vi "Stringhandling (SubVI).vi"(0 "Slide (Eingang)":refnum<vi>, 1 "Füllstand Lesepuffer (Eingang)":i32, 2 "Datei COM (Eingang)":refnum<file>, 3 "VISA-Referenz (Eingang)":refnum<visa-resource-name>, 4 "MessFrequenz [Hz] (Eingang)":dbl, 5 "Bytes at Port":u32, 6 "Datei LV (Eingang)":refnum<file>, 7 "Fehler (Eingang, kein Fehler)":errorcluster, 8 "Cyclecounter (Eingang)":i32, 9 "Rolle[Hz] (Eingang)":dbl, 10 "Temp[°C] (Eingang)":dbl, 11 "AFR (Eingang)":dbl, 12 "String (Eingang)":string, 13 "Zündung [Hz] (Eingang)":dbl) -> (14 "Lesepuffer":string="\n", 16 "Füllstand Lesepuffer (Ausgang)":i32, 17 "String (Ausgang)":string, 18 "Temp[°C] (Ausgang)":dbl, 19 "AFR (Ausgang)":dbl, 20 "VISA-Referenz (Ausgang)":refnum<visa-resource-name>, 21 "Zündung [Hz] (Ausgang)":dbl, 23 "Rolle [Hz] (Ausgang)":dbl, 24 "Messfrequenz [Hz] (Ausgang)":dbl, 25 "Cyclecounter (Ausgang)":i32, 27 "Fehler (Ausgang)":errorcluster)   [LabVIEW 2014]
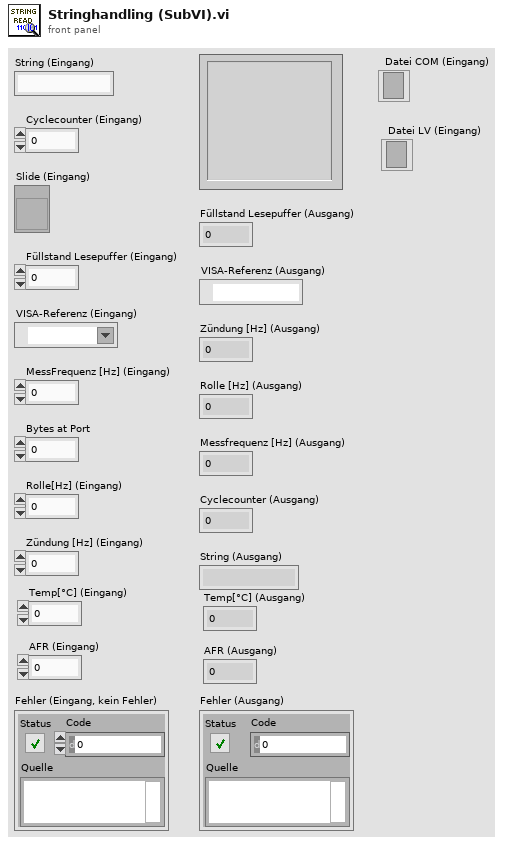
[diagram p1: front panel]
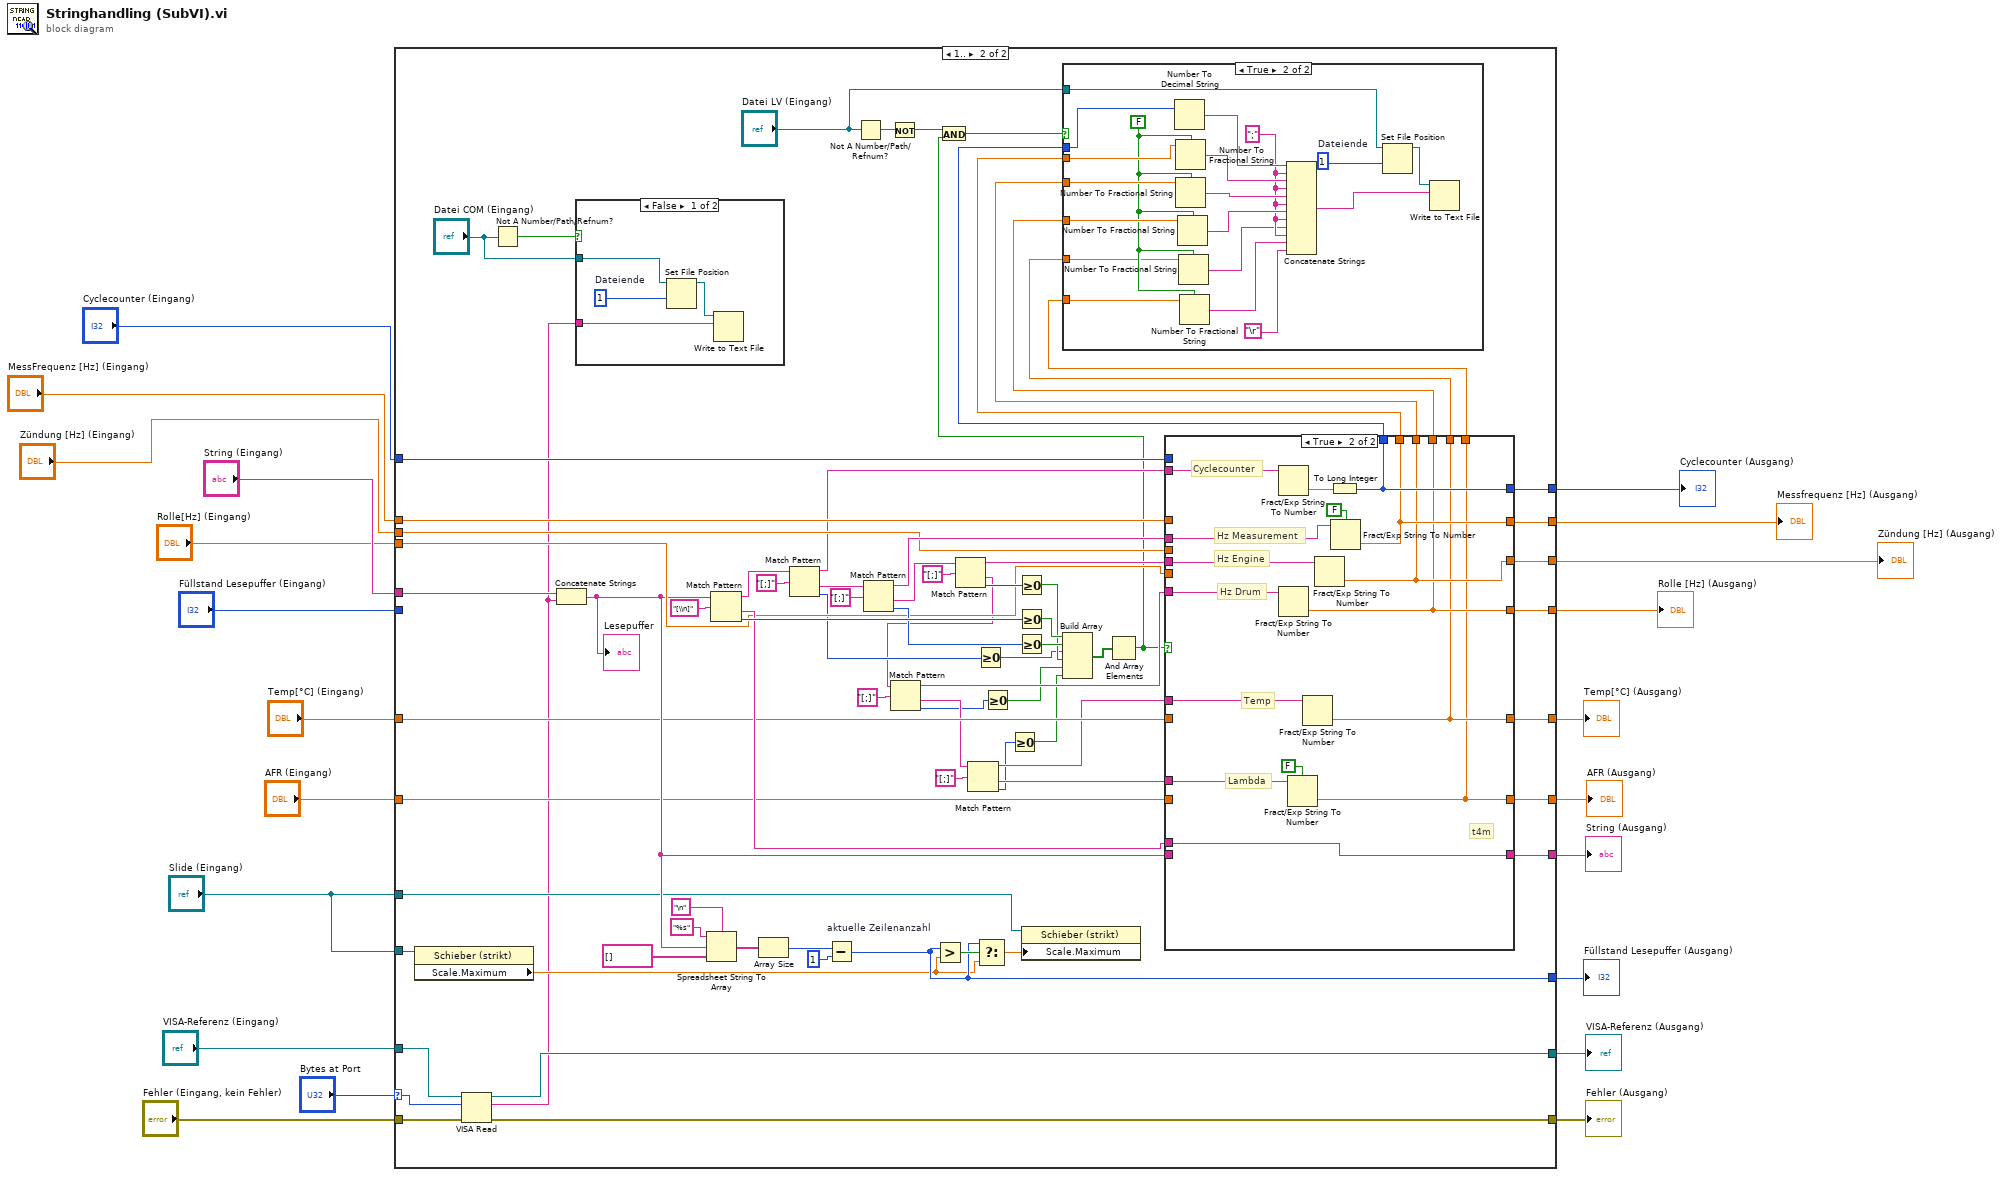
[diagram p0: block diagram]
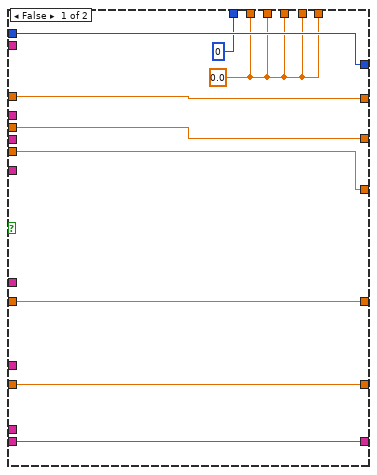
[diagram p5: hidden frame]
diagram:
  n1 = case shown="1.." "Bytes at Port" {
    selector: "Bytes at Port" -> [_ w104]
    tunnel: [w26 w99] -> w14
    tunnel: [w25 w100] -> w19
    tunnel: [w30 w101] -> w12
    tunnel: [w31 w98] -> w11
    tunnel: "String (Eingang)" -> [w32 w97]
    tunnel: [w32 w95] -> w6
    tunnel: "Zündung [Hz] (Eingang)" -> [w31 w88]
    tunnel: "Rolle[Hz] (Eingang)" -> [w30 w87]
    tunnel: [w27 w86] -> w15
    tunnel: "MessFrequenz [Hz] (Eingang)" -> [w27 w85]
    tunnel: "Füllstand Lesepuffer (Eingang)" -> [w29 _]
    tunnel: [w29 w68] -> w13
    tunnel: [w28 w74] -> w16
    tunnel: "Cyclecounter (Eingang)" -> [w28 w73]
    tunnel: "VISA-Referenz (Eingang)" -> [w25 w65]
    tunnel: "Fehler (Eingang, kein Fehler)" -> [w26 w64]
    tunnel: "Slide (Eingang)" -> [_ w63]
    tunnel: "Slide (Eingang)" -> [_ w62]
    tunnel: "Temp[°C] (Eingang)" -> [w24 w61]
    tunnel: [w24 w60] -> w3
    tunnel: [w23 w59] -> w2
    tunnel: "AFR (Eingang)" -> [w23 w58]
    frame 0, Default {
      # "No data in from serial port - Nothing to do."
    }
    frame 1.. {
      n2 = property on="Eigenschaftsknoten" class="Schieber (strikt)"(reference=w63) -> ("Scale.Maximum"=w67:dbl)  [unwired: 1 in, 2 out]
      n3 = VISA Read(VISA resource name=w65, byte count=w104, error in (no error)=w64) -> (VISA resource name out=w100:refnum<visa-resource-name>, read buffer=w45:string, error out=w99:errorcluster)  [unwired: 1 out]
      n4 = Not A Number/Path/Refnum?(number/path/refnum="Datei COM (Eingang)") -> (NaN/Path/Refnum?=w46:bool)
      n5 = Concatenate Strings(w97, w45) -> (w70:string)
      "Lesepuffer" <- w70
      n6 = case shown="False" w46 {
        tunnel: w45 -> [w130 _]
        tunnel: "Datei COM (Eingang)" -> [w129 _]
        frame False {
          w132 = 1  # Dateiende
          n7 = Set File Position(refnum=w129, from (0:start)=w132) -> (refnum out=w131:refnum<file>)  [unwired: 2 in, 1 out]
          n8 = Write to Text File(file (use dialog)=w131, text=w130) -> ()  [unwired: 2 in, 3 out]
        }
        frame True {
        }
      }
      n9 = Spreadsheet String To Array(delimiter (Tab)="\n" ("regular expression"), format string="%s" ("regular expression"), spreadsheet string=w70, array type (2D Dbl)=string[] [] ("Array 2")) -> (array=w79:string[])
      n10 = Match Pattern(string=w70, regular expression="[\\n]") -> (before substring=w77:string, after substring=w96:string, offset past match=w108:i32)  [unwired: 1 in, 1 out]
      n11 = Array Size(array=w79) -> (size(s)=w83:i32)
      n12 = Match Pattern(string=w77, regular expression="[;]") -> (before substring=w75:string, after substring=w76:string, offset past match=w72:i32)  [unwired: 1 in, 1 out]
      n13 = Subtract "aktuelle Zeilenanzahl"(x=w83, y=1) -> (x-y=w68:i32)
      n14 = Not A Number/Path/Refnum?(number/path/refnum="Datei LV (Eingang)") -> (NaN/Path/Refnum?=w34:bool)
      n15 = Match Pattern(string=w76, regular expression="[;]") -> (before substring=w103:string, after substring=w106:string, offset past match=w93:i32)  [unwired: 1 in, 1 out]
      n16 = Not(x=w34) -> (.not. x?=w33:bool)
      n17 = Greater?(x=w68, y=w67) -> (0:w69:bool)
      n18 = Match Pattern(string=w106, regular expression="[;]") -> (before substring=w102:string, after substring=w47:string, offset past match=w91:i32)  [unwired: 1 in, 1 out]
      n19 = Match Pattern(string=w47, regular expression="[;]") -> (before substring=w55:string, after substring=w54:string, offset past match=w49:i32)  [unwired: 1 in, 1 out]
      n20 = Match Pattern(string=w54, regular expression="[;]") -> (before substring=w53:string, after substring=w52:string, offset past match=w48:i32)  [unwired: 1 in, 1 out]
      n21 = Greater Or Equal To 0?(x=w72) -> (x >= 0?=w71:bool)
      n22 = Select(t=w68, s=w69, f=w67) -> (s? t:f=w66:dbl)
      n23 = Greater Or Equal To 0?(x=w49) -> (x >= 0?=w51:bool)
      n24 = Greater Or Equal To 0?(x=w48) -> (x >= 0?=w50:bool)
      n25 = Greater Or Equal To 0?(x=w91) -> (x >= 0?=w90:bool)
      n26 = Greater Or Equal To 0?(x=w108) -> (x >= 0?=w94:bool)
      n27 = Greater Or Equal To 0?(x=w93) -> (x >= 0?=w92:bool)
      n28 = property on="Eigenschaftsknoten" class="Schieber (strikt)"(reference=w62, "Scale.Maximum"=w66) -> ()  [unwired: 1 in, 2 out]
      n29 = Build Array(w94, w92, w71, w90, w51, w50) -> (w89:bool[])
      n30 = And Array Elements(Boolean array=w89) -> (logical AND=w35:bool)
      n31 = And(x=w33, y=w35) -> (x .and. y?=w36:bool)
      n32 = case shown="True" w35 {
        tunnel: w103 -> [_ w154]
        tunnel: w102 -> [_ w157]
        tunnel: w55 -> [_ w156]
        tunnel: [w139 w145] -> w101
        tunnel: [w140 w146] -> w98
        tunnel: w96 -> [_ w155]
        tunnel: [w141 w155] -> w95
        tunnel: w70 -> [w141 _]
        tunnel: w88 -> [w140 _]
        tunnel: w87 -> [w139 _]
        tunnel: [w138 w147] -> w86
        tunnel: w85 -> [w138 _]
        tunnel: w75 -> [_ w153]
        tunnel: [w137 w148] -> w74
        tunnel: w73 -> [w137 _]
        tunnel: w61 -> [w136 _]
        tunnel: [w136 w144] -> w60
        tunnel: [w135 w143] -> w59
        tunnel: w58 -> [w135 _]
        tunnel: w53 -> [_ w151]
        tunnel: w52 -> [_ w150]
        tunnel: [0 w148] -> w42
        tunnel: [w134 w147] -> w39
        tunnel: [w134 w146] -> w41
        tunnel: [w134 w145] -> w40
        tunnel: [w134 w144] -> w38
        tunnel: [w134 w143] -> w37
        frame False {
          w134 = 0.0
        }
        frame True {
          # "Temp"
          # "Lambda"
          # "Cyclecounter"
          # "Hz Measurement"
          # "Hz Drum"
          # "Hz Engine"
          # "t4m"
          n33 = Fract/Exp String To Number(string=w153) -> (number=w152:dbl)  [unwired: 3 in, 1 out]
          n34 = Fract/Exp String To Number(string=w156) -> (number=w145:dbl)  [unwired: 3 in, 1 out]
          n35 = Fract/Exp String To Number(use system decimal point (T)=FALSE, string=w150) -> (number=w143:dbl)  [unwired: 2 in, 1 out]
          n36 = Fract/Exp String To Number(string=w151) -> (number=w144:dbl)  [unwired: 3 in, 1 out]
          n37 = Fract/Exp String To Number(string=w157) -> (number=w146:dbl)  [unwired: 3 in, 1 out]
          n38 = To Long Integer(number=w152) -> (32bit integer=w148:i32)
          n39 = Fract/Exp String To Number(use system decimal point (T)=FALSE, string=w154) -> (number=w147:dbl)  [unwired: 2 in, 1 out]
        }
      }
      n40 = case shown="True" w36 {
        tunnel: "Datei LV (Eingang)" -> [_ w121]
        tunnel: w42 -> [_ w120]
        tunnel: w39 -> [_ w119]
        tunnel: w41 -> [_ w118]
        tunnel: w40 -> [_ w117]
        tunnel: w38 -> [_ w111]
        tunnel: w37 -> [_ w110]
        frame False {
        }
        frame True {
          w127 = 1  # Dateiende
          w116 = ";"
          w115 = FALSE
          n41 = Number To Decimal String(number=w120) -> (decimal integer string=w122:string)  [unwired: 1 in]
          n42 = Number To Fractional String(use system decimal point (T)=w115, number=w119) -> (F-format string=w123:string)  [unwired: 2 in]
          n43 = Number To Fractional String(use system decimal point (T)=w115, number=w118) -> (F-format string=w124:string)  [unwired: 2 in]
          n44 = Number To Fractional String(use system decimal point (T)=w115, number=w117) -> (F-format string=w125:string)  [unwired: 2 in]
          n45 = Number To Fractional String(use system decimal point (T)=w115, number=w111) -> (F-format string=w114:string)  [unwired: 2 in]
          n46 = Number To Fractional String(use system decimal point (T)=w115, number=w110) -> (F-format string=w113:string)  [unwired: 2 in]
          n47 = Concatenate Strings(w122, w116, w123, w116, w124, w116, w125, w116, w114, w116, w113, "\r") -> (w126:string)
          n48 = Set File Position(refnum=w121, from (0:start)=w127) -> (refnum out=w128:refnum<file>)  [unwired: 2 in, 1 out]
          n49 = Write to Text File(file (use dialog)=w128, text=w126) -> ()  [unwired: 2 in, 3 out]
        }
      }
    }
  }
  "VISA-Referenz (Ausgang)" <- w19
  "Cyclecounter (Ausgang)" <- w16
  "Messfrequenz [Hz] (Ausgang)" <- w15
  "Fehler (Ausgang)" <- w14
  "Füllstand Lesepuffer (Ausgang)" <- w13
  "Rolle [Hz] (Ausgang)" <- w12
  "Zündung [Hz] (Ausgang)" <- w11
  "String (Ausgang)" <- w6
  "AFR (Ausgang)" <- w2
  "Temp[°C] (Ausgang)" <- w3
